vi "Set Argument - String Array.vi"(7 "Function Name":string, 8 "Error In":errorcluster, 9 "String Array":string[](array[string]), 10 "Argument":string, 11 "OPI Ref":refnum<data-value>) -> (0 "Error Out":errorcluster, 3 "OPI Ref":refnum<data-value>)   [LabVIEW 2012, in "OPI.lvclass"]
doc: "Set string array argument value for the future function call specified by Function Name.\n\nThe value is transmitted to the PES. This optimizes the speed with which calls can be made, because no data needs to be transmitted at call time."
uses:
  OPI.lvclass
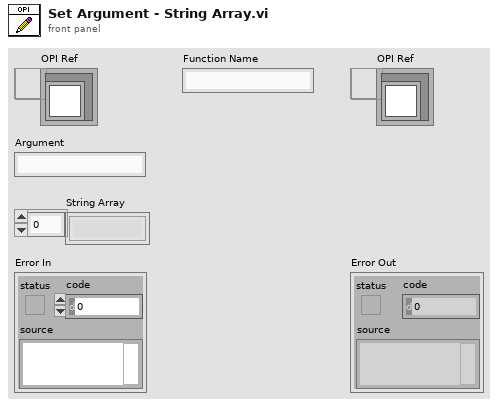
[diagram p1: front panel]
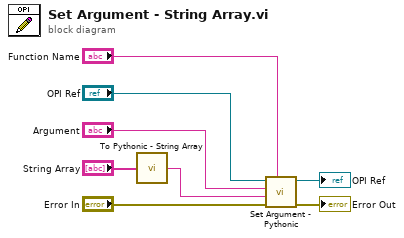
[diagram p0: block diagram]
diagram:
  n1 = call "To Pythonic - String Array.vi"("String Array"="String Array") -> ("Pythonic Value"=w1:string)  [unwired: 4 in]
  n2 = call "Set Argument - Pythonic.vi"("Function Name"="Function Name", "Error In"="Error In", "Pythonic Value"=w1, "Argument"="Argument", "OPI Ref"="OPI Ref") -> ("Error Out"=→"Error Out":errorcluster, "OPI Ref"=→"OPI Ref":refnum<data-value>)  [unwired: 5 in]
